vi "Write Custom Glyph Definitions.vi"(10 "Custom Glyph Definitions":T1[](array[typedef]), 11 "File Explorer in":refnum<class "File Explorer.lvclass">) -> (3 "File Explorer out":refnum<class "File Explorer.lvclass">)   [LabVIEW 2020, in "File Explorer.lvlib" / "File Explorer.lvclass"]
uses:
  <vilib>/gpm_packages/@cs/file-explorer-extension/Source/File Explorer/File Explorer/File Explorer.lvclass
  <vilib>/gpm_packages/@cs/file-explorer-extension/Source/File Explorer/File Explorer/Custom Glyph Definition.ctl
  <vilib>/picture/picture.llb/imagedata.ctl
  <vilib>/gpm_packages/@cs/file-explorer-extension/Source/File Explorer/File Explorer/File Explorer.lvclass/File Explorer.ctl
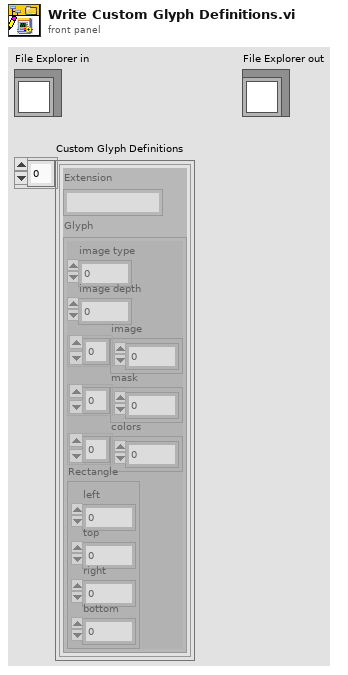
[diagram p1: front panel]
types:
  T1 = typedef "File Explorer.lvlib/File Explorer.lvclass/Custom Glyph Definition.ctl" = cluster{"Extension":string, "Glyph":T2}
  T2 = typedef "imagedata.ctl" = cluster{"image type":i32, "image depth":i32, "image":u8[], "mask":u8[], "colors":u32[], "Rectangle":cluster{"left":i16, "top":i16, "right":i16, "bottom":i16}}
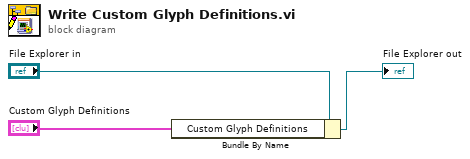
[diagram p0: block diagram]
diagram:
  n1 = Bundle By Name(cluster="File Explorer in", "Custom Glyph Definitions"="Custom Glyph Definitions") -> (→"File Explorer out":refnum<class "File Explorer.lvclass">)
